vi "9103SeriesSetChart.vi"() -> ()   [LabVIEW 2019]
uses:
  <instrlib>/9103Series/9103Series.lvlib
panel:
  in  "Current Setting":dbl(slide) scale=0.0..20.0
  in  "Voltage Setting":dbl(slide) scale=0.0..42.0
  out "error out":errorcluster
  out "CV Mode?":bool
  out "Current":dbl(graph)
  out "Voltage":dbl(graph)
  in  "stop":bool
  in  "VISA resource name":refnum<visa-resource-name>
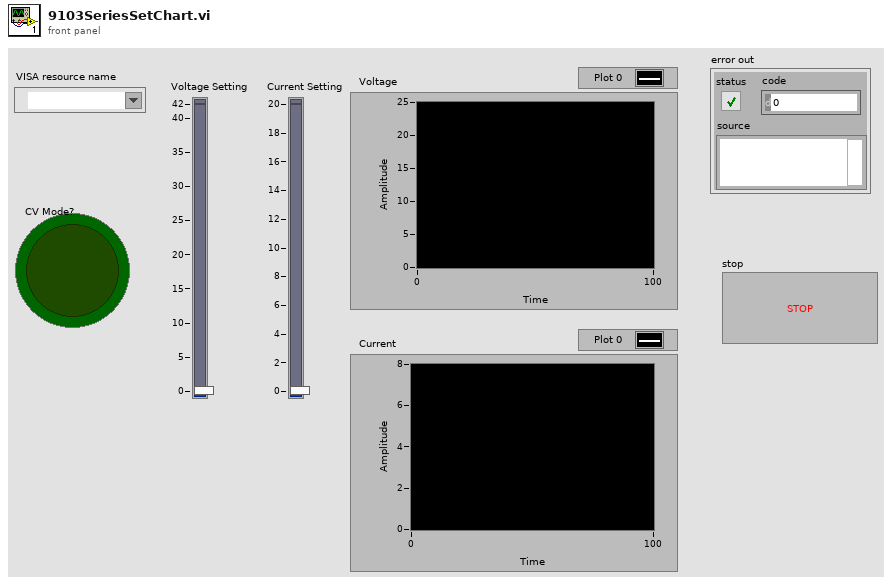
[diagram p1: front panel]
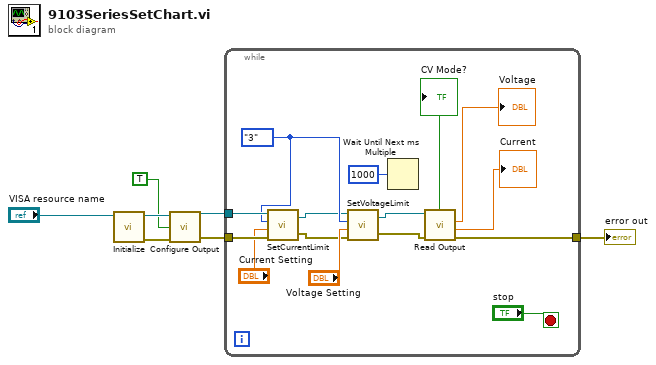
[diagram p0: block diagram]
diagram:
  n1 = call <instrlib>:"Initialize.vi"("VISA resource name"="VISA resource name") -> ("error out"=w7:errorcluster, "VISA resource name out"=w6:refnum<visa-resource-name>)  [unwired: 9 in]
  n2 = call <instrlib>:"Configure Output.vi"("error in (no error)"=w7, "Output On"=TRUE, "VISA resource name"=w6) -> ("error out"=w2:errorcluster, "VISA resource name out"=w3:refnum<visa-resource-name>)  [unwired: 1 in]
  n3 = while {
    tunnel: w3 -> [w13]
    tunnel: w2 -> [w12]
    tunnel: [w17] -> w1
    stop <- "stop" stop-if-true
    w11 = enum16{"0", "1", "2", "3", ""}."3" ("Preset")
    n4 = call <instrlib>:"SetCurrentLimit.vi"("error in (no error)"=w12, "Current"="Current Setting", "Preset"=w11, "VISA resource name"=w13) -> ("error out"=w8:errorcluster, "VISA resource name out"=w9:refnum<visa-resource-name>)
    n5 = call <instrlib>:"SetVoltageLimit.vi"("error in (no error)"=w8, "Voltage"="Voltage Setting", "Preset"=w11, "VISA resource name"=w9) -> ("error out"=w15:errorcluster, "VISA resource name out"=w16:refnum<visa-resource-name>)
    n6 = Wait Until Next ms Multiple(millisecond multiple=u32 1000) -> ()  [unwired: 1 out]
    n7 = call <instrlib>:"Read Output.vi"("error in (no error)"=w15, "VISA resource name"=w16) -> ("error out"=w17:errorcluster, "Current"=→"Current":dbl, "Voltage"=→"Voltage":dbl, "CV Mode?"=→"CV Mode?":bool)  [unwired: 2 in, 1 out]
  }
  "error out" <- w1
